vi "Check Step Complete.vi"(6 "Move Complete":bool, 11 "Main Array in":T1={"FIFO Array"=[{"Auto States"=enum."Initilize", "Dist"=4.3, "Radians"=0.0, "MaxSpeed (ft/s)"=1.2, "TimeOut (s)"=10.0, "CMD"="", "ArmSetpoints"=enum."ShoulderRest"}], "Dist (ft)"=0.0, "MaxSpeed (ft/s)"=0.0, "TimeOut (s)"=99.0, "Timer Value"=0, "DriveStraightDistance"=[], "ModuleTravelPosition"=[0.0, 0.0, 0.0, 0.0], "First Time"=FALSE, "Current Step"={"Auto States"=enum."Unknown", "Dist"=4.3, "Radians"=0.0, "MaxSpeed (ft/s)"=1.2, "TimeOut (s)"=10.0, "CMD"="", "ArmSetpoints"=enum."ShoulderRest"}}) -> (3 "Main Array iout":T1={"FIFO Array"=[{"Auto States"=enum."Initilize", "Dist"=4.3, "Radians"=0.0, "MaxSpeed (ft/s)"=1.2, "TimeOut (s)"=10.0, "CMD"="", "ArmSetpoints"=enum."ShoulderRest"}], "Dist (ft)"=0.0, "MaxSpeed (ft/s)"=0.0, "TimeOut (s)"=99.0, "Timer Value"=0, "DriveStraightDistance"=[], "ModuleTravelPosition"=[0.0, 0.0, 0.0, 0.0], "First Time"=FALSE, "Current Step"={"Auto States"=enum."Unknown", "Dist"=4.3, "Radians"=0.0, "MaxSpeed (ft/s)"=1.2, "TimeOut (s)"=10.0, "CMD"="", "ArmSetpoints"=enum."ShoulderRest"}})   [LabVIEW 2023]
uses:
  Auton Main Array.ctl
  State Machine/FIFO Array.ctl
  State Machine/Auot FIFO.ctl
  State Machine/Auot States.ctl
  Shoulder/ShoulderGetSetpointEnum.ctl
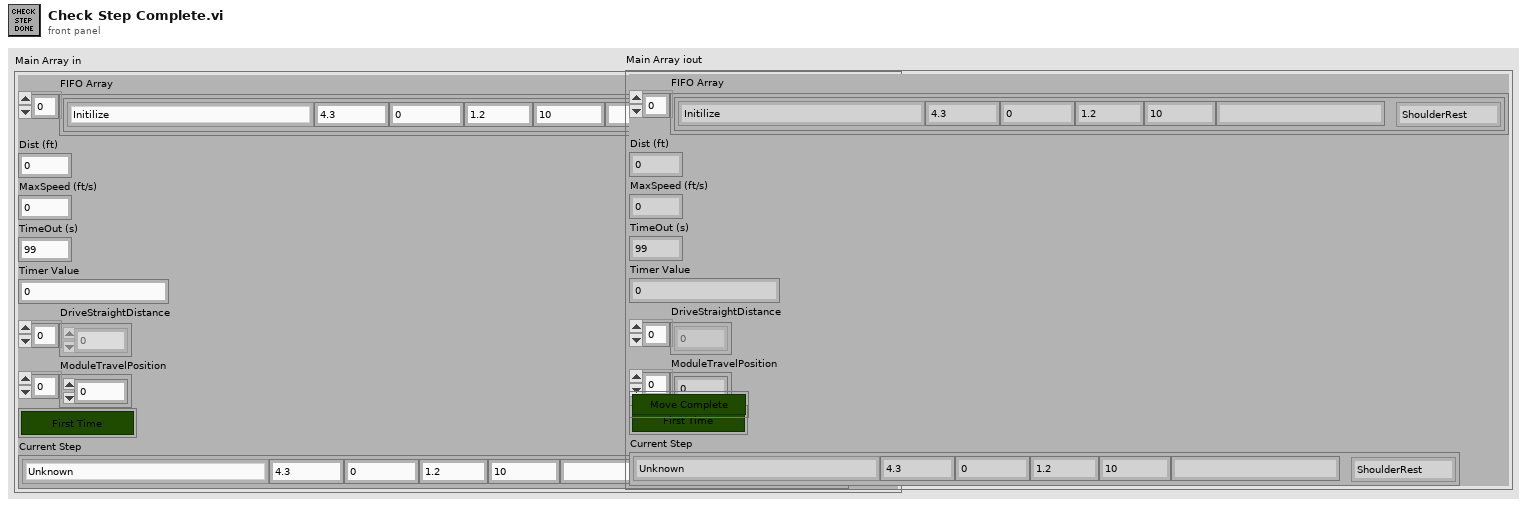
[diagram p1: front panel]
types:
  T1 = typedef "Auton Main Array.ctl" = cluster{"FIFO Array":T2, "Dist (ft)":dbl, "MaxSpeed (ft/s)":dbl, "TimeOut (s)":dbl, "Timer Value":u32, "DriveStraightDistance":dbl[], "ModuleTravelPosition":dbl[], "First Time":bool, "Current Step":T3}
  T2 = typedef "FIFO Array.ctl" = T3[]
  T3 = typedef "Auot FIFO.ctl" = cluster{"Auto States":T4, "Dist":dbl, "Radians":dbl, "MaxSpeed (ft/s)":dbl, "TimeOut (s)":dbl, "CMD":string, "ArmSetpoints":T5}
  T4 = typedef "Auot States.ctl" = enum16{"Unknown", "Initilize", "Intake", "Move Arm", "Drive Straight", "Drive Trajorctory", "Drive Turn", "Send Bool CMD", "Set Target", "Shoot", "Wait", "Exit"}
  T5 = typedef "ShoulderGetSetpointEnum.ctl" = enum16{"Select", "ShoulderRest", "ShoulderSpeaker", "ShoulderAmp"}
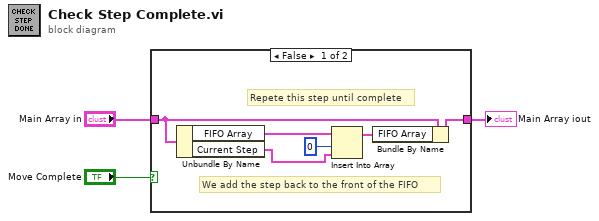
[diagram p0: block diagram]
diagram:
  n1 = case shown="False" "Move Complete" {
    tunnel: "Main Array in" -> [w7 w10]
    tunnel: [w5 w10] -> w1
    frame False {
      # "We add the step back to the front of the FIFO"
      # "Repete this step until complete"
      n2 = Unbundle By Name(w7) -> ("FIFO Array"=w9:T2, "Current Step"=w4:T3)
      n3 = Insert Into Array(array=w9, index=0, new element=w4) -> (w6:T2)
      n4 = Bundle By Name(cluster=w7, "FIFO Array"=w6) -> (w5:T1)
    }
    frame True {
      # "Move on to the next step"
    }
  }
  "Main Array iout" <- w1
